vi "_test_formattingJUnitFromResult.vi"() -> ()   [LabVIEW 2013, in "Caraya.lvlib" / "Test Report.JUnit.lvclass"]
uses:
  Test Report.JUnit.lvclass
  Test Result/Node Results (Extended).ctl
  Test Result/Test Node (Extended).ctl
  Test Result/Test Registration Data.ctl
  Test Result/Assert Event Data (Extended).ctl
  MsgSerializer.XML/MsgSerializer.XML.lvclass
  MsgSerializer.XML/format -- enum.ctl
  MsgSerializer.XML/MsgSerializer.XML.lvclass/MsgSerializer.XML.ctl
  Test Result/Test Result.lvclass
panel:
  out "testcases":string[](array[string])
  in  "testsuites":T1[](array[typedef])
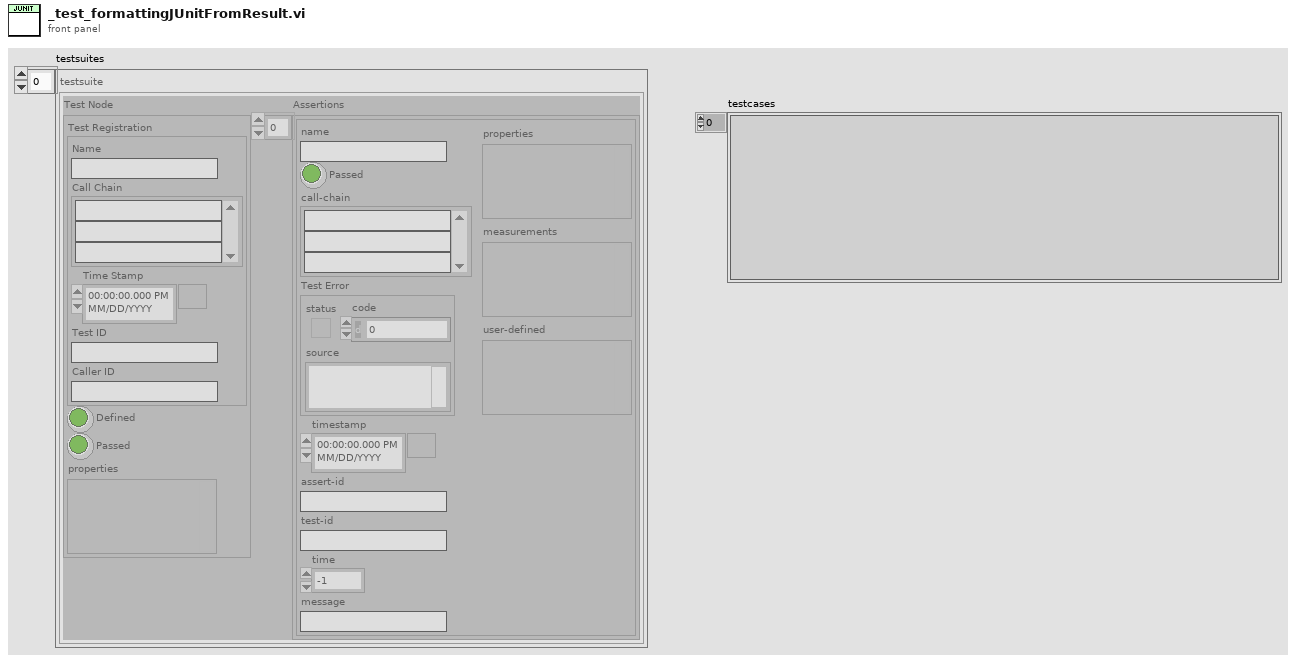
[diagram p1: front panel]
types:
  T1 = typedef "Caraya.lvlib/Test Result.lvclass/Node Results (Extended).ctl" = cluster{"Test Node":T2, "Assertions":T4[]}
  T2 = typedef "Caraya.lvlib/Test Result.lvclass/Test Node (Extended).ctl" = cluster{"Test Registration":T3, "Defined":bool, "Passed":bool, "properties":variant}
  T3 = typedef "Caraya.lvlib/Test Result.lvclass/Test Registration Data.ctl" = cluster{"Name":string, "Call Chain":string[], "Time Stamp":timestamp, "Test ID":string, "Caller ID":string}
  T4 = typedef "Caraya.lvlib/Test Result.lvclass/Assert Event Data (Extended).ctl" = cluster{"name":string, "Passed":bool, "call-chain":string[], "Test Error":errorcluster, "timestamp":timestamp, "assert-id":string, "test-id":string, "time":dbl, "message":string, "properties":variant, "measurements":variant, "user-defined":variant}
  T5 = typedef "Caraya.lvlib/MsgSerializer.XML.lvclass/format -- enum.ctl" = enum16{"value", "tag", "property"}
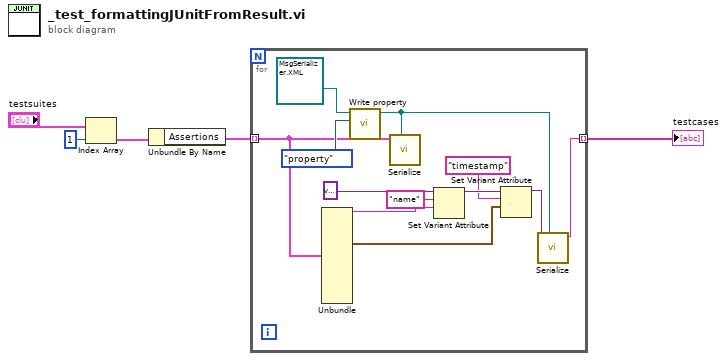
[diagram p0: block diagram]
diagram:
  n1 = Index Array(array="testsuites", index=1) -> (element=w3:T1)
  n2 = Unbundle By Name(w3) -> ("Assertions"=w2:T4[])
  n3 = for {
    tunnel: w2 -> [w15] mode=indexing
    tunnel: [w8] -> w1 mode=indexing
    n4 = Unbundle(w15) -> ("name"=w14:string, "timestamp"=w11:timestamp)  [unwired: 10 out]
    n5 = call "Write property.vi"("format"=format_--_enum."property", "MsgSerializer.XMLProperty in"=refnum<class "MsgSerializer.XML.lvclass"> refnum ("Caraya.lvlib:MsgSerializer.XML.lvclass")) -> ("MsgSerializer.XMLProperty out"=w6:refnum<class "MsgSerializer.XML.lvclass">)  [unwired: 9 in]
    n6 = call-dynamic "Serialize.vi"("MsgSerializer"=w6, "Value"=w15) -> ()  [unwired: 8 in, 2 out]
    n7 = Set Variant Attribute(Variant=variant ("variant"), name="name", value=w14) -> (Variant out=w12:variant)  [unwired: 1 in, 2 out]
    n8 = Set Variant Attribute(Variant=w12, name="timestamp", value=w11) -> (Variant out=w9:variant)  [unwired: 1 in, 2 out]
    n9 = call-dynamic "Serialize.vi"("MsgSerializer"=w6, "Value"=w9) -> ("Serialized Message"=w8:string)  [unwired: 8 in, 1 out]
  }
  "testcases" <- w1
